vi "upload_udc_values.vi"(1 "Transfer Bar":refnum<vi>, 2 "Value Array":dbl[](array[numeric]), 3 "UDC Table":string[][](array[string])) -> ()   [LabVIEW 2011]
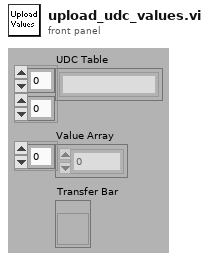
[diagram p1: front panel]
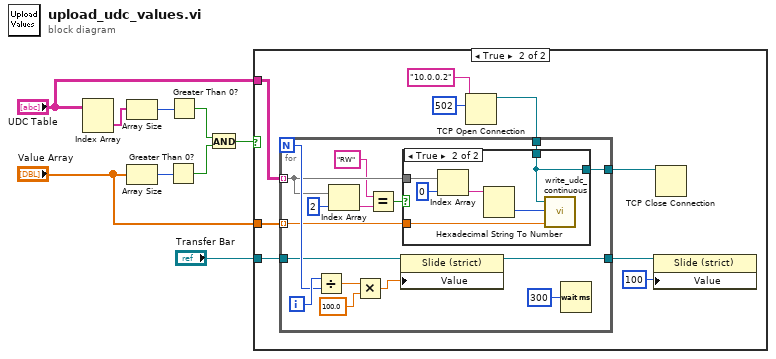
[diagram p0: block diagram]
diagram:
  n1 = Index Array(array="UDC Table") -> (element=w8:string[])  [unwired: 2 in]
  n2 = Array Size(array=w8) -> (size(s)=w9:i32)
  n3 = Array Size(array="Value Array") -> (size(s)=w7:i32)
  n4 = Greater Than 0?(x=w7) -> (x > 0?=w5:bool)
  n5 = Greater Than 0?(x=w9) -> (x > 0?=w6:bool)
  n6 = And(x=w6, y=w5) -> (x .and. y?=w4:bool)
  n7 = case shown="True" w4 {
    tunnel: "UDC Table" -> [_ w18]
    tunnel: "Transfer Bar" -> [_ w17]
    tunnel: "Value Array" -> [_ w11]
    frame False {
    }
    frame True {
      n8 = TCP Open Connection(address="10.0.0.2", remote port or service name=u16 502) -> (connection ID=w12:refnum<k5>)  [unwired: 1 in, 3 out]
      n9 = for {
        N -> [w33]
        tunnel: w18 -> [w25] mode=indexing
        tunnel: w17 -> [w30]
        tunnel: [w28] -> w16
        tunnel: w12 -> [w26]
        tunnel: w11 -> [w27] mode=indexing
        tunnel: [w20] -> w10
        i -> [w34]
        n10 = Divide(x=w34, y=w33) -> (x/y=w32:dbl)
        n11 = Index Array(array=w25, index=2) -> (element=w22:string)
        n12 = Multiply(x=w32, y=100.0) -> (x*y=w29:dbl)
        n13 = Equal?(x="RW", y=w22) -> (x = y?=w23:bool)
        n14 = property class="Slide (strict)"(reference=w30, "Value"=w29) -> (reference out=w28:refnum<vi>)  [unwired: 1 in, 1 out]
        n15 = case shown="True" w23 {
          tunnel: w25 -> [_ w41]
          tunnel: w27 -> [_ w37]
          tunnel: w26 -> [w35 w36]
          tunnel: [w35 w36] -> w20
          frame False {
          }
          frame True {
            n16 = Index Array(array=w41, index=0) -> (element=w39:string)
            n17 = Hexadecimal String To Number(string=w39) -> (number=w38:u32)  [unwired: 3 out]
            n18 = call "write_udc_continuous.vi"("Value"=w37, "Hex Address"=w38, "TCP Connection Refnum in"=w36) -> ()  [unwired: 1 out]
          }
        }
        n19 = Wait (ms)(milliseconds to wait=u32 300) -> ()  [unwired: 1 out]
      }
      n20 = property class="Slide (strict)"(reference=w16, "Value"=u8 100) -> ()  [unwired: 1 in, 2 out]
      n21 = TCP Close Connection(connection ID=w10) -> ()  [unwired: 1 in, 3 out]
    }
  }
